vi "BNC Switch.vi"(8 "error in":errorcluster, 10 "BNC command":string(combo)="BNCoff", 11 "Pressure Box COM":refnum<visa-resource-name>) -> (0 "error out":errorcluster, 2 "Response":string, 3 "Pressure Box COM out":refnum<visa-resource-name>)   [LabVIEW 2015]
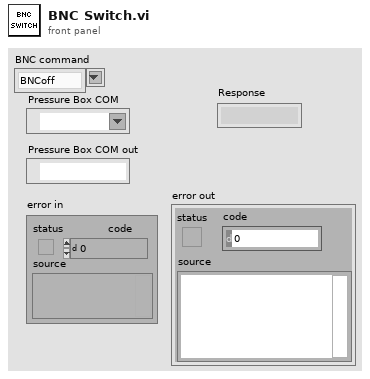
[diagram p1: front panel]
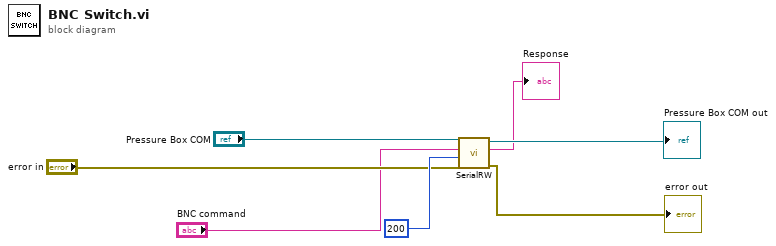
[diagram p0: block diagram]
diagram:
  n1 = call "SerialRW.vi"("error in (no error)"="error in", "Delay (ms)"=u32 200, "Command"="BNC command", "VISA handle"="Pressure Box COM") -> ("error out"=→"error out":errorcluster, "Response"=→"Response":string, "Dup. VISA handle"=→"Pressure Box COM out":refnum<visa-resource-name>)  [unwired: 2 in, 1 out]
